vi "clear Session Data.vi"(0 "Session in":refnum<class "VariableContainer.lvclass">, 11 "error in":errorcluster) -> (4 "Session out":refnum<class "VariableContainer.lvclass">, 15 "error out":errorcluster)   [LabVIEW 2020, in "HTS.lvlib" / "VariableContainer.lvclass"]
uses:
  VariableContainer.lvclass
  VariableContainer.lvclass/VariableContainer.ctl
  <userlib>/_Session Fwk/Session - Root.lvclass
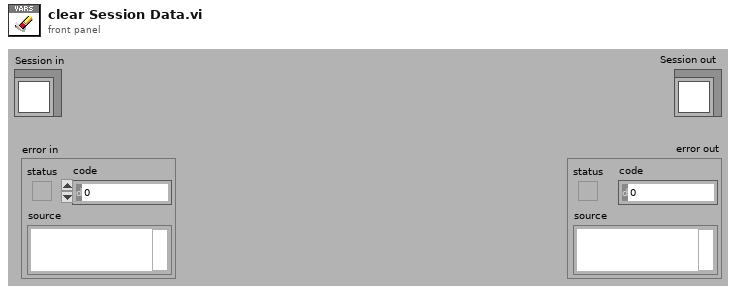
[diagram p1: front panel]
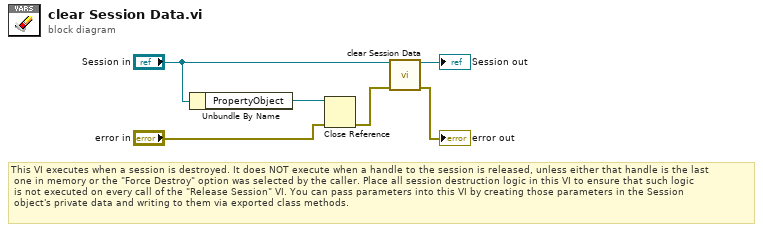
[diagram p0: block diagram]
diagram:
  # "This VI executes when a session is destroyed. It does NOT execute when a handle to the session is released, unless either that handle is the last\n one in memory or the \"Force Destroy\" option was selected by the caller. Place all session destruction logic in this VI to ensure that such logic\n is not executed on every call of the \"Release Session\" VI. You can pass parameters into this VI by creating those parameters in the Session \n object's private data and writing to them via exported class methods."
  n1 = Unbundle By Name("Session in") -> ("PropertyObject"=w1:refnum<k7>)
  n2 = Close Reference(reference=w1, error in (no error)="error in") -> (error out=w2:errorcluster)
  n3 = call-parent "clear Session Data.vi"("OBJ - Measurement Session in"="Session in", "error in"=w2) -> ("OBJ - Measurement Session out"=→"Session out":refnum<class "VariableContainer.lvclass">, "error out"=→"error out":errorcluster)  [unwired: 12 in]
